vi "ConfigUtilities - Get Rx Packet Information.vi"(8 "error in (no error)":errorcluster, 11 "Device Item Ref in":T1 format="%.0x") -> (0 "error out":errorcluster, 2 "Array":T2[](array[typedef]), 3 "Device Item Ref out":T1 format="%.0x")   [LabVIEW 2015, in "UDP-Custom-Device System Explorer.lvlib"]
uses:
  UDP-Custom-Device System Explorer.lvlib
  Shared/Rx.PacketInfo.ctl
  <vilib>/NI Veristand/Custom Device API/Custom Device Item Ref.ctl
  Shared/Constants.vi
  <vilib>/NI Veristand/Custom Device API/Get Item Property (I32 Array).vi
  <vilib>/NI Veristand/Custom Device API/Get Item Property (String Array).vi
  Shared/UDP-Custom-Device Shared.lvlib
  <vilib>/NI VeriStand/Custom Device API/Custom Device API.lvlib
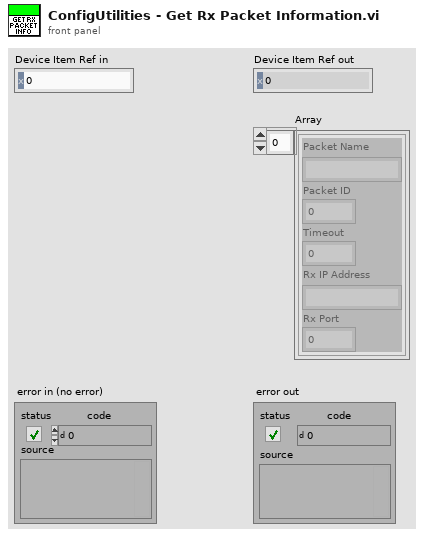
[diagram p1: front panel]
types:
  T1 = typedef "Custom Device API.lvlib/Custom Device Item Ref.ctl" = u64
  T2 = typedef "UDP-Custom-Device Shared.lvlib/Rx.PacketInfo.ctl" = cluster{"Packet Name":string, "Packet ID":i32, "Timeout":i32, "Rx IP Address":string, "Rx Port":i32}
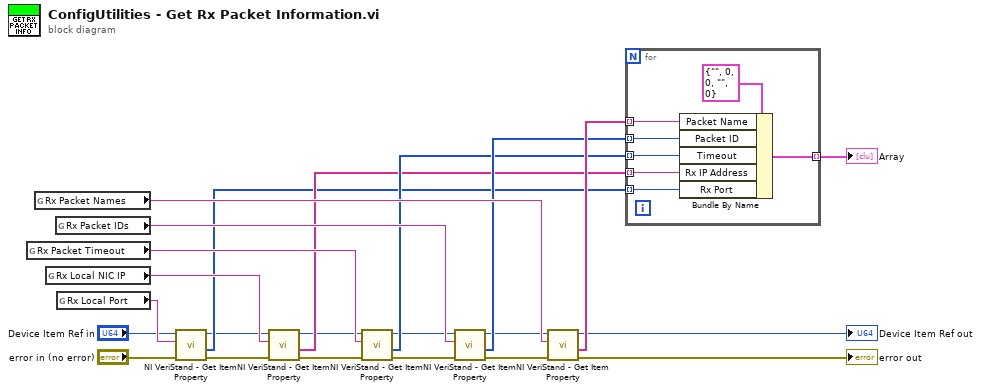
[diagram p0: block diagram]
diagram:
  n1 = global read "Constants.vi" "Rx Packet Timeout"() -> (w20:string)
  n2 = global read "Constants.vi" "Rx Packet Names"() -> (w18:string)
  n3 = global read "Constants.vi" "Rx Local NIC IP"() -> (w21:string)
  n4 = global read "Constants.vi" "Rx Packet IDs"() -> (w19:string)
  n5 = global read "Constants.vi" "Rx Local Port"() -> (w22:string)
  n6 = call-poly <vilib>:"NI VeriStand - Get Item Property.vi"("error in (no error)"="error in (no error)", "Property Name"=w22, "Item Ref in"="Device Item Ref in") -> ("error out"=w7:errorcluster, "Value"=w12:i32[], "Item Ref out"=w11:T1)  [unwired: 5 in, 1 out]
  n7 = call-poly <vilib>:"NI VeriStand - Get Item Property.vi"("error in (no error)"=w7, "Property Name"=w21, "Item Ref in"=w11) -> ("error out"=w6:errorcluster, "Value"=w13:string[], "Item Ref out"=w10:T1)  [unwired: 5 in, 1 out]
  n8 = call-poly <vilib>:"NI VeriStand - Get Item Property.vi"("error in (no error)"=w6, "Property Name"=w20, "Item Ref in"=w10) -> ("error out"=w5:errorcluster, "Value"=w14:i32[], "Item Ref out"=w9:T1)  [unwired: 5 in, 1 out]
  n9 = call-poly <vilib>:"NI VeriStand - Get Item Property.vi"("error in (no error)"=w5, "Property Name"=w19, "Item Ref in"=w9) -> ("error out"=w4:errorcluster, "Value"=w15:i32[], "Item Ref out"=w8:T1)  [unwired: 5 in, 1 out]
  n10 = call-poly <vilib>:"NI VeriStand - Get Item Property.vi"("error in (no error)"=w4, "Property Name"=w18, "Item Ref in"=w8) -> ("error out"=→"error out":errorcluster, "Value"=w16:string[], "Item Ref out"=→"Device Item Ref out":T1)  [unwired: 5 in, 1 out]
  n11 = for {
    tunnel: w16 -> [w29] mode=indexing
    tunnel: w15 -> [w28] mode=indexing
    tunnel: w14 -> [w27] mode=indexing
    tunnel: w13 -> [w26] mode=indexing
    tunnel: w12 -> [w25] mode=indexing
    tunnel: [w24] -> w2 mode=indexing
    n12 = Bundle By Name(cluster=T2 {"Packet Name"="", "Packet ID"=0, "Timeout"=0, "Rx IP Address"="", "Rx Port"=0} ("Packet Info"), "Packet Name"=w29, "Packet ID"=w28, "Timeout"=w27, "Rx IP Address"=w26, "Rx Port"=w25) -> (w24:T2)
  }
  "Array" <- w2
